vi "error generator.vi"(8 "error in":errorcluster, 9 "source":string="Error Cluster From Error Code.vi", 10 "append error message":string, 11 "error code (0)":i32) -> (0 "error out":errorcluster)   [LabVIEW 2013, in "TBM configuration.lvclass"]
doc: "Converts an error or warning code to an error cluster. This VI is useful when you receive a return value from a shared library call or when you return user-defined error codes."
uses:
  TBM configuration.lvclass
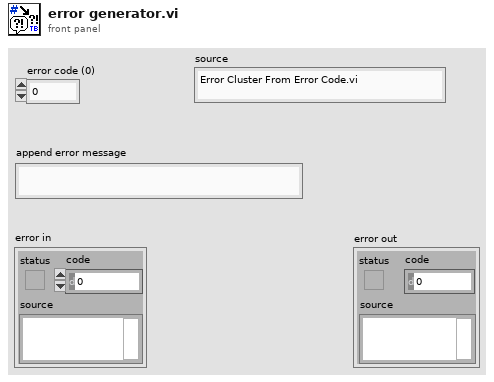
[diagram p1: front panel]
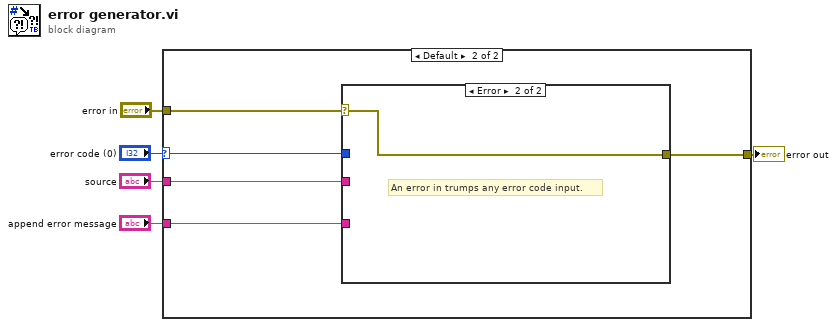
[diagram p0: block diagram]
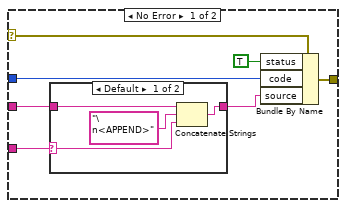
[diagram p3: hidden frame]
diagram:
  n1 = case shown="Default" "error code (0)" {
    selector: "error code (0)" -> [_ w9]
    tunnel: "error in" -> [w6 w11]
    tunnel: [w6 w10] -> w3
    tunnel: "source" -> [_ w8]
    tunnel: "append error message" -> [_ w7]
    frame 0 {
      # "If the error code in equals zero, then propagate the error in cluster regardless of its value."
    }
    frame Default {
      n2 = case shown="Error" w11 {
        selector: w11 -> [w16 w24]
        tunnel: [w17 w24] -> w10
        tunnel: w9 -> [w18 _]
        tunnel: w8 -> [w12 _]
        tunnel: w7 -> [w14 _]
        frame No Error {
          n3 = case shown="Default" w14 {
            selector: w14 -> [w20 _]
            tunnel: [w19 w23] -> w13
            tunnel: w12 -> [w22 w23]
            frame Default {
              n4 = Concatenate Strings(w22, "\n<APPEND>" ("string"), w20) -> (w19:string)
            }
            frame "" {
            }
          }
          n5 = Bundle By Name(cluster=w16, "status"=TRUE, "code"=w18, "source"=w13) -> (w17:errorcluster)
        }
        frame Error {
          # "An error in trumps any error code input."
        }
      }
    }
  }
  "error out" <- w3
